vi "TSLIN SetMapping.vi"(0 "路径输入":path, 5 "LINCount":i32(ring)=1 items=["1通道"=1, "2通道"=2, "3通道"=3, "4通道"=4, "5通道"=5], 7 "Tsapp_setLIN_mapping_verbose_Type":T1(array[cluster]) {"AProtocol" items=["Lin_Protocol_13", "Lin_Protocol_20", "Lin_Protocol_21", "Lin_Protocol_J2602"]; "AArbRateKbps" format="%#_g  k"; "AEnableMapping" items=["Disable", "Enable"]; "AAppChannelType" items=["APP_CAN", "APP_LIN"]; "AHardwareChannel" items=["CHN1", "CHN2", "CHN3", "CHN4", "CHN5", "CHN6", "CHN7", "CHN8", "CHN9", "CHN10", "CHN11", "CHN12", "CHN13", "CHN14", "CHN15", "CHN16", "CHN17", "CHN18", "CHN19", "CHN20", "CHN21", "CHN22", "CHN23", "CHN24", "CHN25", "CHN26", "CHN27", "CHN28", "CHN29", "CHN30", "CHN31", "CHN32"]; "AAppChannel" items=["CHN1", "CHN2", "CHN3", "CHN4", "CHN5", "CHN6", "CHN7", "CHN8", "CHN9", "CHN10", "CHN11", "CHN12", "CHN13", "CHN14", "CHN15", "CHN16", "CHN17", "CHN18", "CHN19", "CHN20", "CHN21", "CHN22", "CHN23", "CHN24", "CHN25", "CHN26", "CHN27", "CHN28", "CHN29", "CHN30", "CHN31", "CHN32"]; "AHardwareType" items=["BUS_UNKNOWN_TYPE", "TS_TCP_DEVICE", "XL_USB_DEVICE", "TS_USB_DEVICE", "PEAK_USB_DEVICE", "KVASER_USB_DEVICE", "ZLG_USB_DEVICE", "ICS_USB_DEVICE", "TS_TC1005_DEVICE"]; "AHardwareSubType" items=["TS_UNKNOWN_DEVICE", "TSCAN_PRO", "TSCAN_Litel", "TC1001", "TL1001", "TC1011", "TSInterface", "TC1002", "TC1014", "TCCANFD2517", "TC1026", "TC1016", "TC1012", "TC1013"]}, 11 "错误输入（无错误）":errorcluster) -> (4 "路径输出":path, 6 "LINCount":i32(ring)=1 items=["1通道"=1, "2通道"=2, "3通道"=3, "4通道"=4, "5通道"=5], 15 "错误输出":errorcluster)   [LabVIEW 2013]
panel:
  out "SetLIN_Baudrated_Successfully":bool[](array[boolean])
  out "MappingLIN_Successfully":bool[](array[boolean])
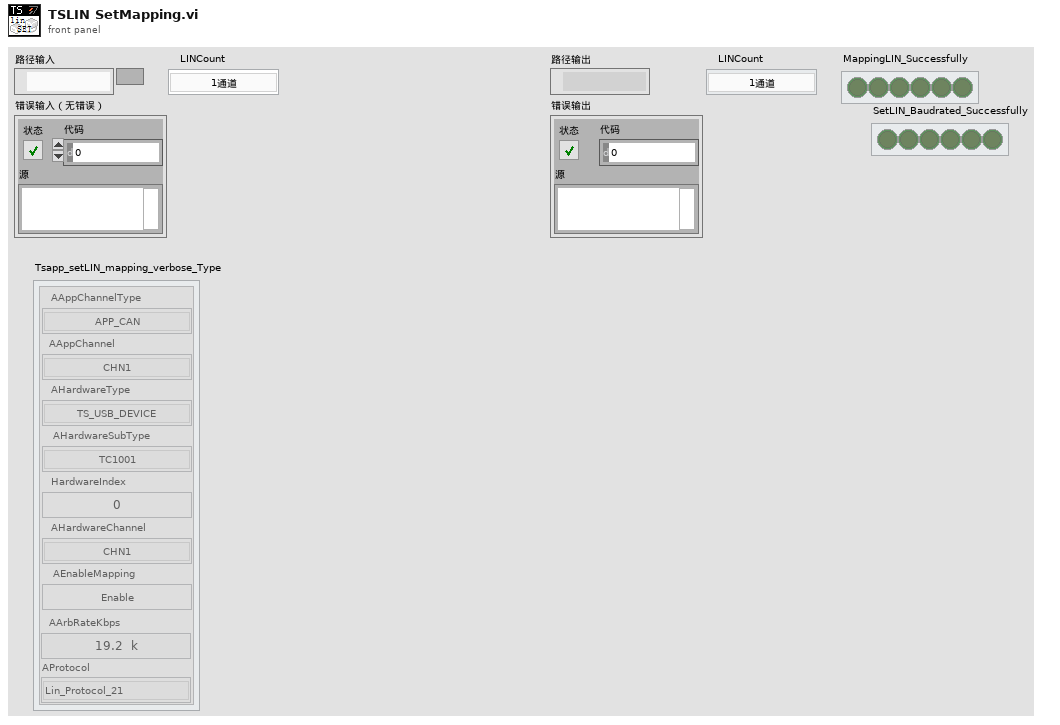
[diagram p1: front panel]
types:
  T1 = cluster{"AAppChannelType":i32, "AAppChannel":i32, "AHardwareType":i32, "AHardwareSubType":i32, "HardwareIndex":i32, "AHardwareChannel":i32, "AEnableMapping":u32, "AArbRateKbps":sgl, "AProtocol":i32}[]
  T2 = cluster{"AAppChannelType":i32, "AAppChannel":i32, "AHardwareType":i32, "AHardwareSubType":i32, "HardwareIndex":i32, "AHardwareChannel":i32, "AEnableMapping":u32, "AArbRateKbps":sgl, "AProtocol":i32}
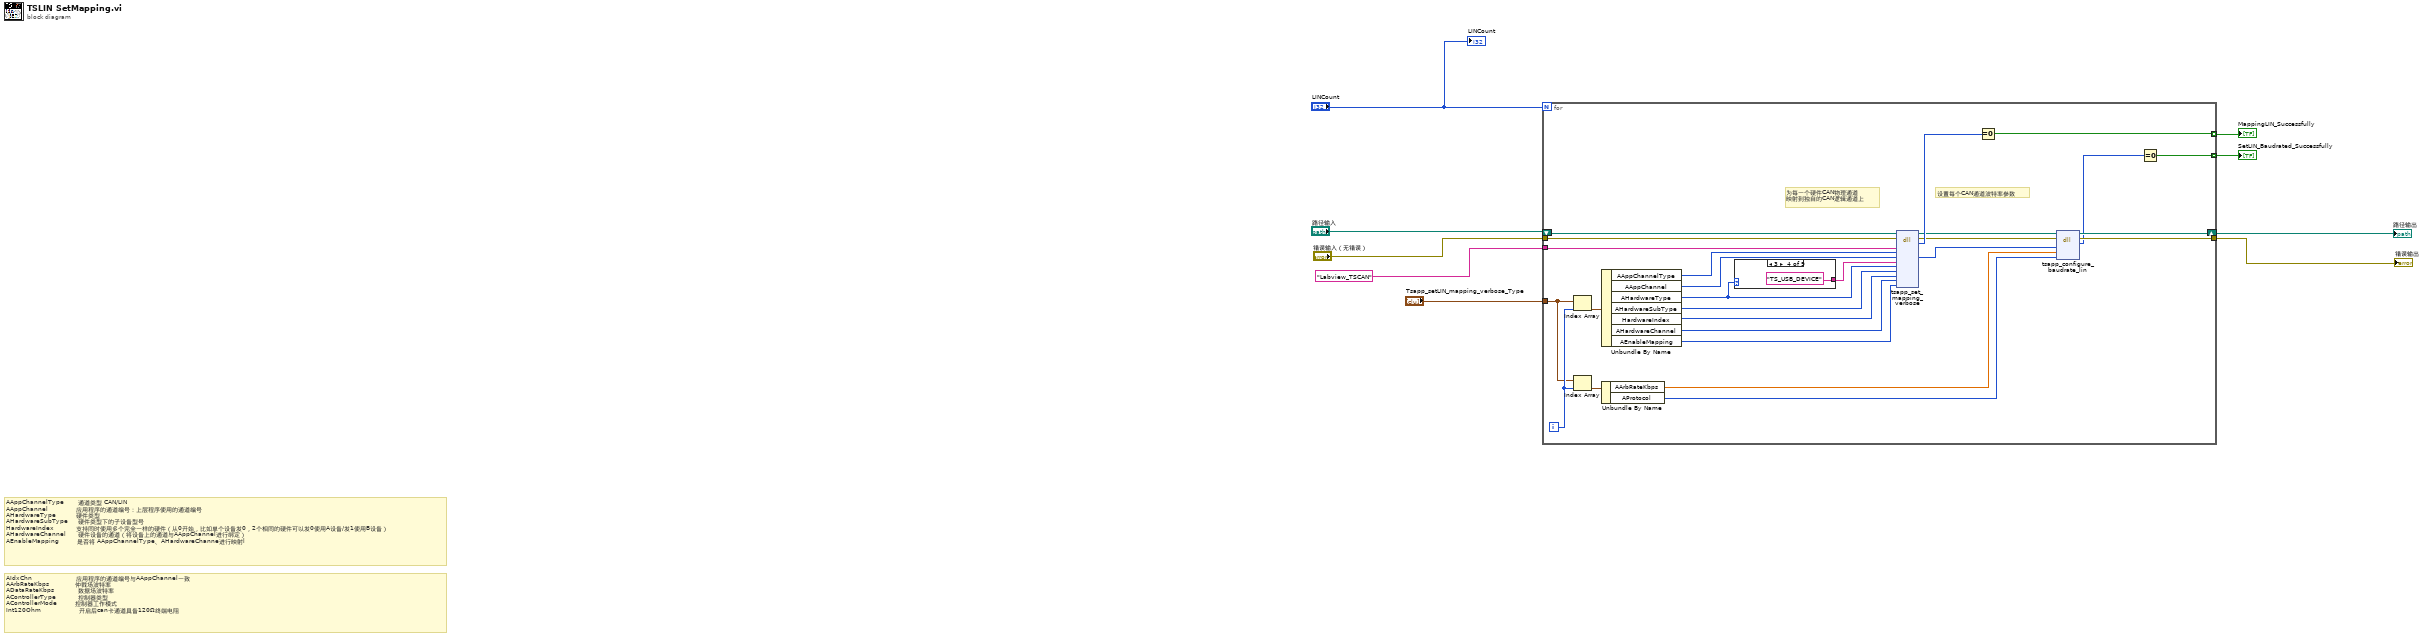
[diagram p0: block diagram]
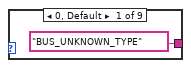
[diagram p2: hidden frame]
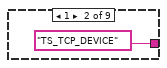
[diagram p3: hidden frame]
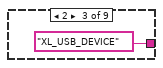
[diagram p4: hidden frame]
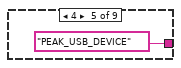
[diagram p5: hidden frame]
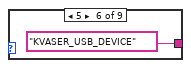
[diagram p6: hidden frame]
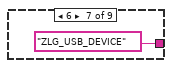
[diagram p7: hidden frame]
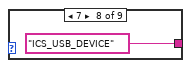
[diagram p8: hidden frame]
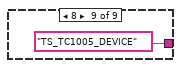
[diagram p9: hidden frame]
diagram:
  # "AIdxChn                      应用程序的通道编号与AAppChannel一致\nAArbRateKbps             仲裁场波特率\nADataRateKbps            数据场波特率\nAControllerType           控制器类型\nAControllerMode         控制器工作模式\nInt120Ohm                   开启后can卡通道具备120Ω终端电阻"
  # "AAppChannelType       通道类型 CAN/LIN\nAAppChannel              应用程序的通道编号：上层程序使用的通道编号\nAHardwareType          硬件类型\nAHardwareSubType     硬件类型下的子设备型号\nHardwareIndex           支持同时使用多个完全一样的硬件（从0开始，比如单个设备发0，2个相同的硬件可以发0使用A设备/发1使用B设备）\nAHardwareChannel      硬件设备的通道（将设备上的通道与AAppChannel进行绑定）\nAEnableMapping         是否将 AAppChannelType、AHardwareChanne进行映射l"
  n1 = for {
    N: "LINCount" -> [_]
    tunnel: "错误输入（无错误）" -> [w32]
    tunnel: "Labview_TSCAN" ("AppName") -> [w31]
    tunnel: "Tsapp_setLIN_mapping_verbose_Type" -> [w10]
    shift-right: [w17] -> w2
    shift-left: "路径输入" -> [w33]
    tunnel: [w16] -> w1
    tunnel: [w22] -> w5 mode=indexing
    tunnel: [w21] -> w4 mode=indexing
    i -> [w20]
    # "设置每个CAN通道波特率参数"
    # "为每一个硬件CAN物理通道\n映射到独自的CAN逻辑通道上"
    n2 = Index Array(array=w10, index=w20) -> (element=w23:T2)
    n3 = Index Array(array=w10, index=w20) -> (element=w13:T2)
    n4 = Unbundle By Name(w13) -> ("AArbRateKbps"=w12:sgl, "AProtocol"=w11:i32)
    n5 = Unbundle By Name(w23) -> ("AAppChannelType"=w30:i32, "AAppChannel"=w29:i32, "AHardwareType"=w28:i32, "AHardwareSubType"=w27:i32, "HardwareIndex"=w26:i32, "AHardwareChannel"=w25:i32, "AEnableMapping"=w24:u32)
    n6 = case shown="3" w28 {
      tunnel: ["BUS_UNKNOWN_TYPE" ("AHardwareName") "TS_TCP_DEVICE" ("AHardwareName") "XL_USB_DEVICE" ("AHardwareName") "TS_USB_DEVICE" ("AHardwareName") "PEAK_USB_DEVICE" ("AHardwareName") "KVASER_USB_DEVICE" ("AHardwareName") "ZLG_USB_DEVICE" ("AHardwareName") "ICS_USB_DEVICE" ("AHardwareName") "TS_TC1005_DEVICE" ("AHardwareName")] -> w35
      frame 0, Default {
      }
      frame 1 {
      }
      frame 2 {
      }
      frame 3 {
      }
      frame 4 {
      }
      frame 5 {
      }
      frame 6 {
      }
      frame 7 {
      }
      frame 8 {
      }
    }
    n7 = dll-call lib="PTH1Habs CUsers\nAdministratorDesktopTS_Can通讯PathTSMaster.dll" fn="tsapp_set_mapping_verbose"(path in=w33, error in=w32, "FAPppName"=w31, "AChnType"=w30, "FAppChannelIndex"=w29, "AHWDeviceName"=w35, "AHWDeviceType"=w28, "AHWDeviceSubType"=w27, "AldHW"=w26, "AldHWChn"=w25, "FMappingDisabled"=w24) -> (path out=w19:path, error out=w18:errorcluster, "tsapp_set_mapping_verbose"=w34:i32, "FAppChannelIndex"=w15:i32)  [unwired: 9 in]
    n8 = Equal To 0?(x=w34) -> (x = 0?=w22:bool)
    n9 = dll-call lib="PTH1@abs EDemo同星TSCAN_V1.4_20220301ConfigTSMaster.dll" fn="tsapp_configure_baudrate_lin"(path in=w19, error in=w18, "ALdxChn"=w15, "ABaudrateKbps"=w12, "AProtocol"=w11) -> (path out=w17:path, error out=w16:errorcluster, "tsapp_configure_baudrate_can"=w14:i32)  [unwired: 4 in]
    n10 = Equal To 0?(x=w14) -> (x = 0?=w21:bool)
  }
  "路径输出" <- w2
  "错误输出" <- w1
  "MappingLIN_Successfully" <- w5
  "SetLIN_Baudrated_Successfully" <- w4
  "LINCount" <- "LINCount"
